vi "SIAM-TMSI.vi"(7 "ResolutionBits-Table":u8[][](array[numeric])=[[20, 20, 16, 16], [20, 20, 16, 16], [20, 20, 16, 16], [20, 20, 16, 16], [12, 12, 8, 8]], 8 "error in (no error)":errorcluster, 9 "use ticket":bool, 10 "Type":enum8{"acc", "vel", "abs", "offset"}(ring), 11 "Motor":T2(ring)) -> (0 "error out":errorcluster, 1 "Ticket":u32 format="%.0x", 2 "Resolution-Factor":i32, 3 "command":T1=4027514895 format="%x" items=["read_x-Motor_status_ticket"=17305600, "init_x-Motor"=17760263, "read_x-Motor_absolute_ticket"=16781312, "move_x-Motor_absolute"=16777217, "move_x-Motor_relative"=16842753, "read_y-Motor_status_ticket"=18354176, "init_y-Motor"=18808839, "read_y-Motor_absolute_ticket"=17829888, "move_y-Motor_absolute"=17825793, "move_y-Motor_relative"=17891329, "read_z-Motor_status_ticket"=19402752, "init_z-Motor"=19857415, "stop_z-Motor"=19857423, "start_z-Motor"=19857422, "read_z-Motor_absolute_ticket"=18878464, "move_z-Motor_absolute"=18874369, "move_z-Motor_relative"=18939905, "end_no_ticket"=4027514895, "end_ticket"=4027518991, "IO-read_bank0"=3489665024, "IO-write_bank0"=3489660929, "IO-read_bank1"=3506442240, "IO-write_bank1"=3506438145, "Analog-write_DA0-0"=2684354561, "Analog-write_DA0-1"=2685403137, "Analog-write_DA0-2"=2686451713, "Analog-write_DA0-3"=2687500289, "Analog-write_DA0-4"=2688548865, "Analog-write_DA0-5"=2689597441, "Analog-write_DA0-6"=2690646017, "Analog-write_DA0-7"=2691694593, "Analog-write_DA1-0"=2701131777, "Analog-write_DA1-1"=2702180353, "Analog-write_DA1-2"=2703228929, "Analog-write_DA1-3"=2704277505, "Analog-write_DA1-4"=2705326081, "Analog-write_DA1-5"=2706374657, "Analog-write_DA1-6"=2707423233, "Analog-write_DA1-7"=2708471809, "Analog-read_AD0-0"=2818576384, "Analog-read-store_AD0-0"=2818572290, "IO-delay_bank0"=3489923073, "IO-delay_bank0_fromVar"=3489923075, "read_cam_clock"=3289124864, "store_cam_clock"=3289120770, "read_cam_phase"=3289190400, "set_cam_deadtime"=3288989697, "set_cam_10uscycles"=3289055233, "set_cam_10uscycles_fromVariable"=3289055235, "calc_cam"=3289317386, "store_cam_Var"=3289251842, "math_addToVariable"=4060086278, "readVar"=4060090368, "writeVar"=4060086273, "copyVar"=4060086276, "decrement_branchRel_if_equal"=4043374945, "decrement_branchRel_if_greaterequal"=4043375201, "decrement_branchRel_if_greaterequal_withTicket"=4043379297, "decrement_branchRel_if_smaller"=4043375457, "increment_branchRel_if_smaller"=4043375473, "set_x-Galvo"=102760689, "set_y-Galvo"=103809265, "set_z-Fokus"=104857841, "set_x-Galvo_position-only"=102760513, "set_y-Galvo_position-only"=103809089, "set_z-Fokus_position-only"=104857665, "set_x-Galvo_position-only_ticket"=102764609, "set_y-Galvo_position-only_ticket"=103813185, "set_z-Fokus_position-only_ticket"=104861761, "set_x-Galvo_speed-only"=102760481, "set_y-Galvo_speed-only"=103809057, "set_z-Fokus_speed-only"=104857633, "read_x-Galvo_ticket"=102764608, "read_y-Galvo_ticket"=103813184, "read_z-Focus_ticket"=104861760, "x-Galvo_pos_fromVar"=102760515, "y-Galvo_pos_fromVar"=103809091, "z-Focus_pos_fromVar"=104857667])   [LabVIEW 2011]
uses:
  SIAM_command.ctl
panel:
  in  "Motor-Ticket-Konstants":u32[](array[numeric])=[0, 0, 0, 0, 512]
  out "2^n":u8
  out "x*2^n":u32 format="%x"
  # "At the moment not all bitmasks are named.\nSo 6x000x1 is unknown but valid command"
  # "Motor# is value in bit20..24"
  # "Type is bitmask bit4..8"
  # "command set and scaling"
  # "dont really store ticket here as there is non-TMSI devices with tickets"
  # "type"
  # "Motor"
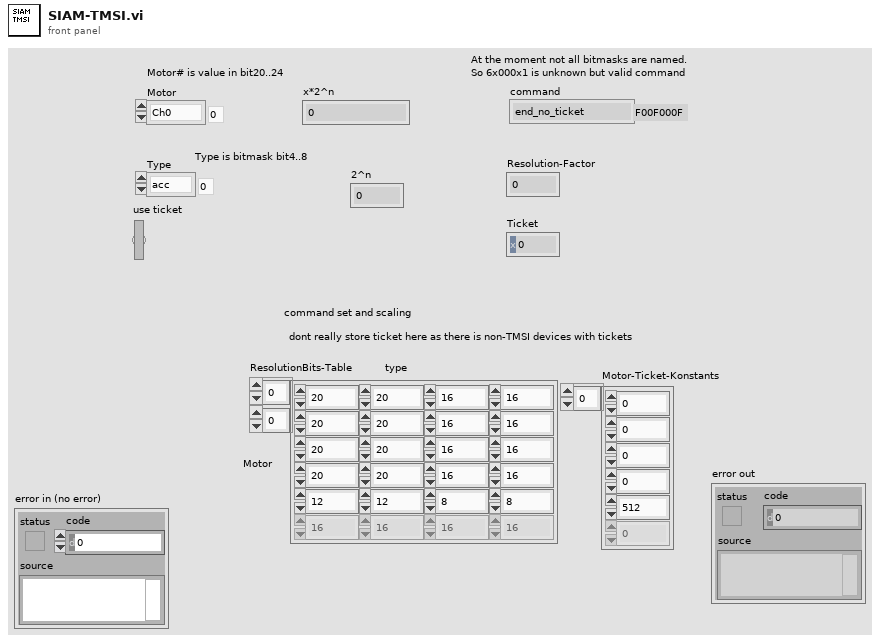
[diagram p1: front panel]
types:
  T1 = typedef "SIAM_command.ctl" = u32
  T2 = enum8{"Ch0", "Ch1", "x-Galvo", "y-Galvo", "z-Focus"}
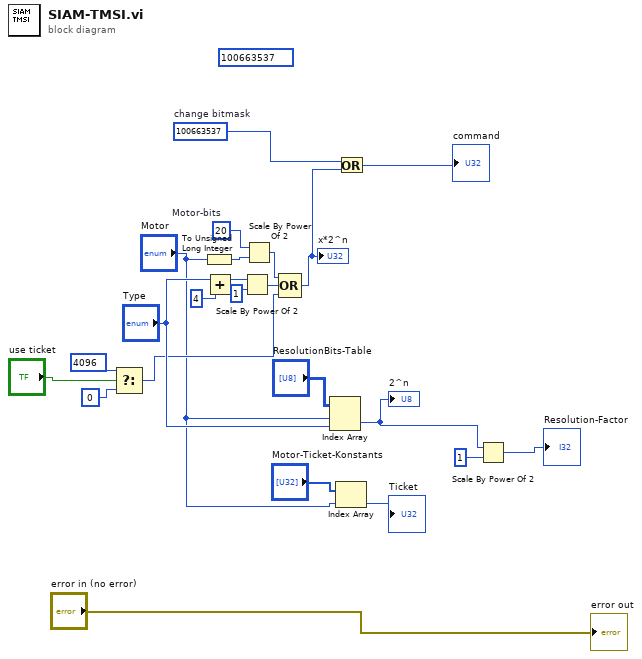
[diagram p0: block diagram]
diagram:
  w1 = u32 100663537  # change bitmask
  w23 = u8 20  # Motor-bits
  (unwired) T1 100663537 items=["read_x-Motor_status_ticket"=17305600, "init_x-Motor"=17760263, "read_x-Motor_absolute_ticket"=16781312, "move_x-Motor_absolute"=16777217, "move_x-Motor_relative"=16842753, "read_y-Motor_status_ticket"=18354176, "init_y-Motor"=18808839, "read_y-Motor_absolute_ticket"=17829888, "move_y-Motor_absolute"=17825793, "move_y-Motor_relative"=17891329, "read_z-Motor_status_ticket"=19402752, "init_z-Motor"=19857415, "stop_z-Motor"=19857423, "start_z-Motor"=19857422, "read_z-Motor_absolute_ticket"=18878464, "move_z-Motor_absolute"=18874369, "move_z-Motor_relative"=18939905, "end_no_ticket"=4027514895, "end_ticket"=4027518991, "IO-read_bank0"=218107904, "IO-write_bank0"=218103809, "IO-read_bank1"=219156480, "IO-write_bank1"=219152385, "IO-delay_bank0"=218365953, "IO-delay_bank0_fromVar"=218365955, "read_cam_clock"=3289124864, "store_cam_clock"=3289120770, "read_cam_phase"=3289190400, "set_cam_deadtime"=3288989697, "set_cam_10uscycles"=3289055233, "set_cam_10uscycles_fromVariable"=3289055235, "calc_cam"=3289317386, "store_cam_Var"=3289251842, "math_addToVariable"=4060086278, "readVar"=4060090368, "writeVar"=4060086273, "copyVar"=4060086276, "decrement_branchRel_if_equal"=4043374945, "decrement_branchRel_if_greaterequal"=4043375201, "decrement_branchRel_if_greaterequal_withTicket"=4043379297, "decrement_branchRel_if_smaller"=4043375457, "increment_branchRel_if_smaller"=4043375473, "set_x-Galvo"=102760689, "set_y-Galvo"=103809265, "set_z-Fokus"=104857841, "read_x-Galvo_ticket"=102764608, "read_y-Galvo_ticket"=103813184, "read_z-Focus_ticket"=104861760, "x-Galvo_pos_fromVar"=102760515, "y-Galvo_pos_fromVar"=103809091, "z-Focus_pos_fromVar"=104857667] ("command 2")
  n1 = Select(t=u32 4096, s="use ticket", f=u32 0) -> (s? t:f=w5:u32)
  n2 = To Unsigned Long Integer(number="Motor") -> (unsigned 32bit integer=w17:u32)
  n3 = Add(x="Type", y=u8 4) -> (x+y=w10:u8)
  n4 = Scale By Power Of 2(n=w10, x=u32 1) -> (x*2^n=w15:u32)
  n5 = Scale By Power Of 2(n=w23, x=w17) -> (x*2^n=w14:u32)
  n6 = Compound Arithmetic op=OR(w14, w15, w5) -> (w13:u32)
  "x*2^n" <- w13
  n7 = Index Array(array="ResolutionBits-Table", index (row)="Motor", index (col)="Type") -> (element=w19:u8)
  "2^n" <- w19
  n8 = Index Array(array="Motor-Ticket-Konstants", index="Motor") -> (element=→"Ticket":u32)
  n9 = Or(x=w1, y=w13) -> (x .or. y?=→"command":u32)
  n10 = Scale By Power Of 2(n=w19, x=1) -> (x*2^n=→"Resolution-Factor":i32)
  "error out" <- "error in (no error)"
